vi "IMU_Global.vi"() -> ()   [LabVIEW 2015]
uses:
  Gyro_TypeDef.ctl
  Accel_TypeDef.ctl
  Mag_TypeDef.ctl
panel:
  in  "Reset_IMU":bool
  out "mag_active":bool
  out "gyro_active":bool
  out "accel_active":bool
  out "Mag":T1
  out "Accel":T2
  out "Gyro":T3
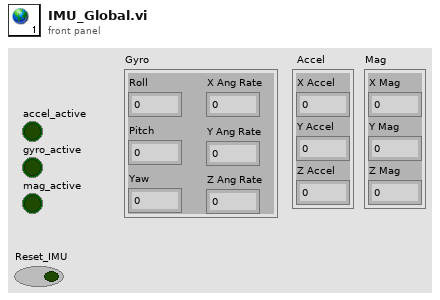
[diagram p1: front panel]
types:
  T1 = typedef "Mag_TypeDef.ctl" = cluster{"X Mag":dbl, "Y Mag":dbl, "Z Mag":dbl}
  T2 = typedef "Accel_TypeDef.ctl" = cluster{"X Accel":dbl, "Y Accel":dbl, "Z Accel":dbl}
  T3 = typedef "Gyro_TypeDef.ctl" = cluster{"Pitch":dbl, "Yaw":dbl, "X Ang Rate":dbl, "Y Ang Rate":dbl, "Z Ang Rate":dbl, "Roll":dbl}
diagram:
